vi "Change State.vi"(8 "error in (no error)":errorcluster, 10 "New State In":refnum<class "State.lvclass">, 11 "Door Controller in":refnum<class "Door Controller.lvclass">) -> (0 "error out":errorcluster, 3 "State Out":refnum<class "State.lvclass">)   [LabVIEW 2020, in "Door Controller.lvlib" / "Door Controller.lvclass"]
uses:
  Door Controller.lvclass
  C:/Program Files/National Instruments/LabVIEW 2020/vi.lib/ActorFramework/Actor/Actor.lvclass
  C:/Users/Thomas.McQuillan/Desktop/Elevator Door Control/State/State.lvclass
  State/State.lvclass
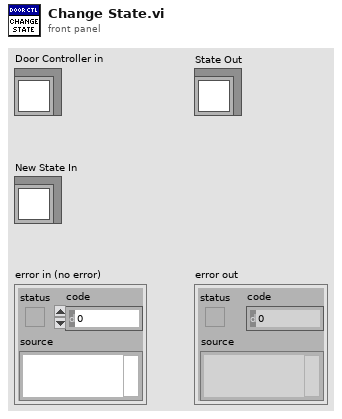
[diagram p1: front panel]
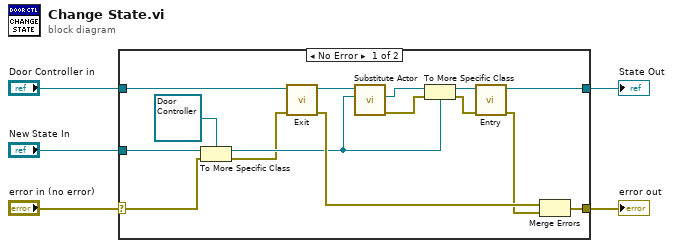
[diagram p0: block diagram]
diagram:
  n1 = case shown="No Error" "error in (no error)" {
    selector: "error in (no error)" -> [w8 w21]
    tunnel: "Door Controller in" -> [w20 w22]
    tunnel: [w19 w22] -> w2
    tunnel: "New State In" -> [w10 _]
    tunnel: [w12 w21] -> w3
    frame No Error {
      n2 = To More Specific Class(target class=refnum<class "Door Controller.lvclass"> refnum ("Door Controller.lvlib:Door Controller.lvclass"), reference=w10, error in=w8) -> (specific class reference=w9:refnum<class "Door Controller.lvclass">, error out=w7:errorcluster)
      n3 = call-dynamic "Exit.vi"("error in (no error)"=w7, "Door Controller in"=w20) -> ("error out"=w14:errorcluster, "Door Controller out"=w18:refnum<class "Door Controller.lvclass">)  [unwired: 8 in]
      n4 = call-dynamic "Substitute Actor.vi"("Substitute Actor in"=w9, "Current Door Controller"=w18) -> ("error out"=w17:errorcluster, "Substitute Actor out"=w16:refnum<class "Actor.lvclass">)  [unwired: 8 in]
      n5 = To More Specific Class(target class=w9, reference=w16, error in=w17) -> (specific class reference=w6:refnum<class "Door Controller.lvclass">, error out=w15:errorcluster)
      n6 = call-dynamic "Entry.vi"("error in (no error)"=w15, "Door Controller in"=w6) -> ("error out"=w13:errorcluster, "Door Controller out"=w19:refnum<class "Door Controller.lvclass">)  [unwired: 8 in]
      n7 = Merge Errors(w14, w13) -> (w12:errorcluster)
    }
    frame Error {
    }
  }
  "error out" <- w3
  "State Out" <- w2
